vi "20220221-main.vi"() -> ()   [LabVIEW 2019]
uses:
  52/sub/state.ctl
  52/sub/servo state.ctl
  20220212-contest/ctl/move.ctl
  ctl/continued move array-V2.ctl
  <vilib>/myRIO/Common/Instrument Driver Framework/myRIO v1.0/UART/vis/myRIO v1.0 Close UART.vi
  <vilib>/myRIO/Common/Instrument Driver Framework/Utilities/vis/FPGA Ref Manager.vi
  <vilib>/myRIO/Common/Instrument Driver Framework/myRIO v1.0/myRIO v1.0 Reset FPGA.vi
  <vilib>/myRIO/Common/Instrument Driver Framework/myRIO v1.0/IRQ/vis/myRIO v1.0 IRQ Info FGV.vi
  <vilib>/myRIO/Common/Instrument Driver Framework/myRIO v1.0/IRQ/vis/myRIO v1.0 Timer IRQ Info FGV.vi
  <vilib>/myRIO/Common/Instrument Driver Framework/myRIO v1.0/IRQ/vis/myRIO v1.0 ISR Agent.vi
  <vilib>/myRIO/Instrument Drivers/Utilities/vis/Reset Index.vi
  <vilib>/myRIO/Common/Instrument Driver Framework/myRIO v1.0/Resource Manager/vis/myRIO v1.0 Block Write Resource Manager.vi
  <vilib>/myRIO/Instrument Drivers/Utilities/Utilities.lvlib
panel:
  out "error out":errorcluster
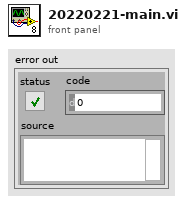
[diagram p1: front panel]
types:
  T1 = typedef "servo state.ctl" = enum16{"catch", "cam-1", "put", "side", "center", "side-2"}
  T2 = typedef "state.ctl" = enum16{"vision", "catch", "recycle", "go home"}
  T3 = typedef "move.ctl" = enum16{"S - box", "box - R1", "R1 - box", "box - R2", "R2 - box", "box - R3", "R3 - box", "box - R4", "R4 - box", "box - R5", "R5 - box", "box - rec", "rec - box", "box - S", "box align", "box end"}
  T4 = typedef "continued move array-V2.ctl" = cluster{"X":dbl, "Y":dbl, "Speed":dbl, "rotate\ndegree":dbl, "deg":dbl}
  T5 = typedef "position cluster.ctl" = cluster{"X":dbl, "Y":dbl, "Angle":dbl}
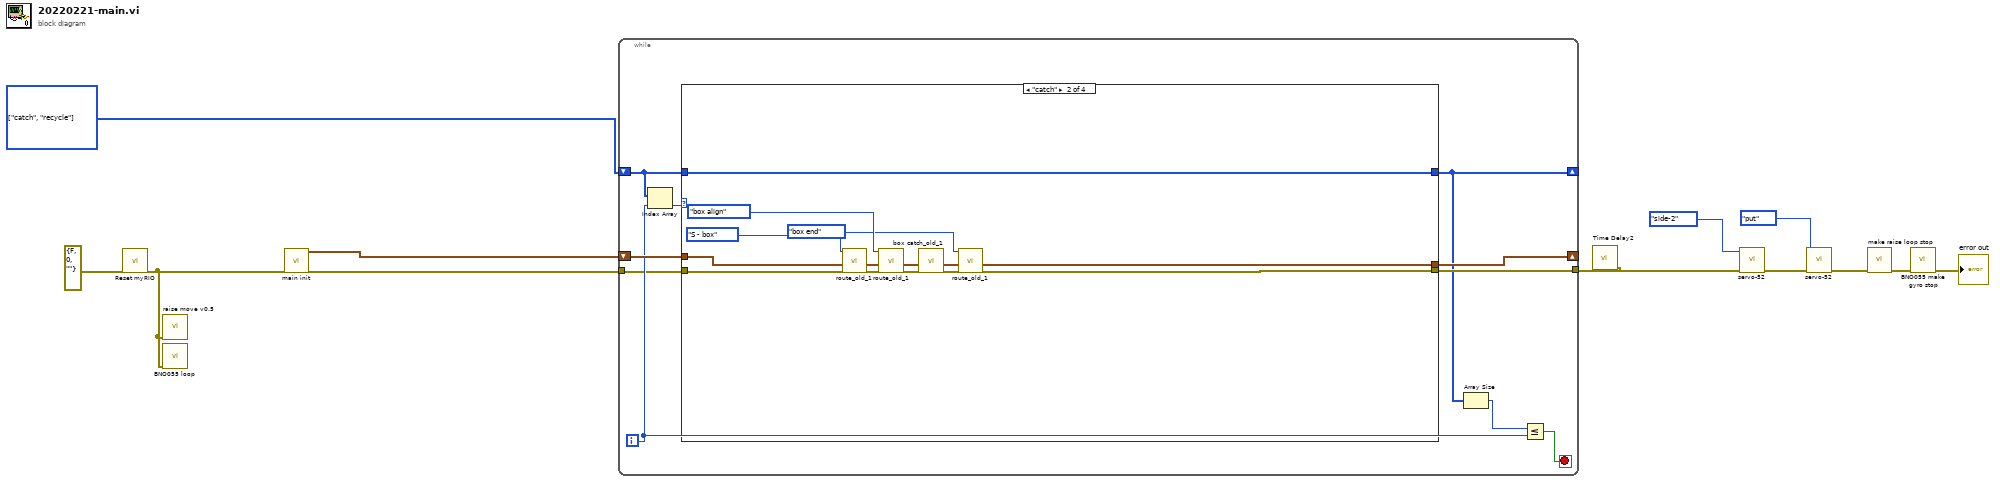
[diagram p0: block diagram]
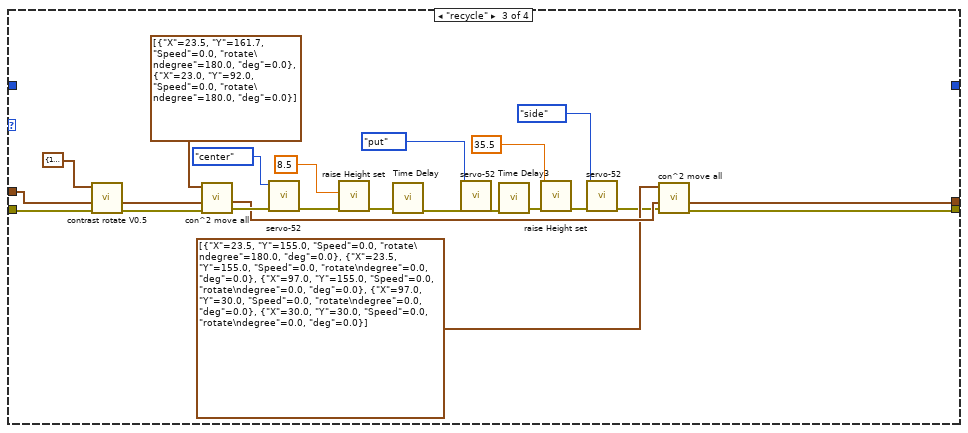
[diagram p3: hidden frame]
diagram:
  w13 = T2[] [enum."catch", enum."recycle"] items=["vision", "catch", "recycle", "go home"]
  n1 = call <vilib>:"Reset myRIO.vi"("error in (no error)"=errorcluster {"status"=FALSE, "code"=0, "source"=""}) -> ("error out"=w3:errorcluster)  [unwired: 10 in]
  n2 = call "raise move v0.5.vi"("error in (no error)"=w3) -> ()  [unwired: 10 in, 1 out]
  n3 = call "BNO055 loop.vi"("error in (no error)"=w3) -> ()  [unwired: 11 in]
  n4 = call "main init.vi"("error in (no error)"=w3) -> ("error out"=w10:errorcluster, "position out"=w9:cluster{"x":dbl, "y":dbl, "degree":dbl})  [unwired: 9 in]
  n5 = while {
    shift-right: [w18] -> _
    shift-left: w13 -> [w22]
    tunnel: [w21] -> w12
    shift-right: [w19] -> _
    shift-left: w9 -> [w20]
    tunnel: w10 -> [w15]
    i -> [w17]
    stop <- w16 stop-if-true
    n6 = Index Array(array=w22, index=w17) -> (element=w23:T2)
    n7 = case shown="\"catch\"" w23 {
      tunnel: w22 -> [_ w39 _ _]
      tunnel: [_ w39 _ _] -> w18
      tunnel: [w25 w26 w47 w64] -> w21
      tunnel: w20 -> [w24 w33 w51 w63]
      tunnel: [w24 w27 w46 w63] -> w19
      tunnel: w15 -> [w25 w35 w52 w64]
      frame "vision", Default {
      }
      frame "catch" {
        n8 = call "route_old_1.vi"("error in (no error)"=w35, "now position"=w33, "Enum"=move."S - box") -> ("error out"=w37:errorcluster, "position out"=w34:cluster{"x":dbl, "y":dbl, "degree":dbl})  [unwired: 7 in]
        n9 = call "route_old_1.vi"("error in (no error)"=w37, "now position"=w34, "Enum"=move."box align") -> ("error out"=w32:errorcluster, "position out"=w31:cluster{"x":dbl, "y":dbl, "degree":dbl})  [unwired: 7 in]
        n10 = call "box catch_old_1.vi"("error in (no error)"=w32, "now position"=w31) -> ("error out"=w30:errorcluster, "position out"=w29:cluster{"x":dbl, "y":dbl, "degree":dbl})  [unwired: 8 in]
        n11 = call "route_old_1.vi"("error in (no error)"=w30, "now position"=w29, "Enum"=move."box end") -> ("error out"=w26:errorcluster, "position out"=w27:cluster{"x":dbl, "y":dbl, "degree":dbl})  [unwired: 7 in]
      }
      frame "recycle" {
        n12 = call "contrast rotate V0.5.vi"("error in (no error)"=w52, "Position in"=w51, "Target Angle"=cluster{"Angle":dbl, "speed":dbl} {"Angle"=180.0, "speed"=80.0}) -> ("error out"=w54:errorcluster, "output cluster"=w53:T5)  [unwired: 7 in]
        n13 = call "con^2 move all.vi"("error in (no error)"=w54, "now position"=w53, "contrast move array"=T4[] [{"X"=23.5, "Y"=161.7, "Speed"=0.0, "rotate\ndegree"=180.0, "deg"=0.0}, {"X"=23.0, "Y"=92.0, "Speed"=0.0, "rotate\ndegree"=180.0, "deg"=0.0}]) -> ("error out"=w60:errorcluster, "position out"=w49:cluster{"x":dbl, "y":dbl, "degree":dbl})  [unwired: 7 in]
        n14 = call "servo-52.vi"("error in (no error)"=w60, "Enum"=servo_state."center") -> ("error out"=w59:errorcluster)  [unwired: 9 in]
        n15 = call "raise Height set.vi"("error in (no error)"=w59, "Height_cm"=8.5) -> ("error out"=w57:errorcluster)  [unwired: 9 in]
        n16 = call "Time Delay"("error in (no error)"=w57) -> ("error out"=w56:errorcluster)  [unwired: 10 in]
        n17 = call "servo-52.vi"("error in (no error)"=w56, "Enum"=servo_state."put") -> ("error out"=w45:errorcluster)  [unwired: 9 in]
        n18 = call "Time Delay3"("error in (no error)"=w45) -> ("error out"=w44:errorcluster)  [unwired: 10 in]
        n19 = call "raise Height set.vi"("error in (no error)"=w44, "Height_cm"=35.5) -> ("error out"=w42:errorcluster)  [unwired: 9 in]
        n20 = call "servo-52.vi"("error in (no error)"=w42, "Enum"=servo_state."side") -> ("error out"=w41:errorcluster)  [unwired: 9 in]
        n21 = call "con^2 move all.vi"("error in (no error)"=w41, "now position"=w49, "contrast move array"=T4[] [{"X"=23.5, "Y"=155.0, "Speed"=0.0, "rotate\ndegree"=180.0, "deg"=0.0}, {"X"=23.5, "Y"=155.0, "Speed"=0.0, "rotate\ndegree"=0.0, "deg"=0.0}, {"X"=97.0, "Y"=155.0, "Speed"=0.0, "rotate\ndegree"=0.0, "deg"=0.0}, {"X"=97.0, "Y"=30.0, "Speed"=0.0, "rotate\ndegree"=0.0, "deg"=0.0}, {"X"=30.0, "Y"=30.0, "Speed"=0.0, "rotate\ndegree"=0.0, "deg"=0.0}]) -> ("error out"=w47:errorcluster, "position out"=w46:cluster{"x":dbl, "y":dbl, "degree":dbl})  [unwired: 7 in]
      }
      frame "go home" {
      }
    }
    n22 = Array Size(array=w18) -> (size(s)=w14:i32)
    n23 = Less Or Equal?(x=w14, y=w17) -> (x <= y?=w16:bool)
  }
  n24 = call "Time Delay2"("error in (no error)"=w12) -> ("error out"=w1:errorcluster)  [unwired: 10 in]
  n25 = call "servo-52.vi"("error in (no error)"=w1, "Enum"=servo_state."side-2") -> ("error out"=w7:errorcluster)  [unwired: 9 in]
  n26 = call "servo-52.vi"("error in (no error)"=w7, "Enum"=servo_state."put") -> ("error out"=w5:errorcluster)  [unwired: 9 in]
  n27 = call "make raise loop stop.vi"("error in (no error)"=w5) -> ("error out"=w8:errorcluster)  [unwired: 10 in]
  n28 = call "BNO055 make gyro stop .vi"("error in (no error)"=w8) -> ("error out"=→"error out":errorcluster)  [unwired: 10 in]
